vi "OSCILO.vi"(4 "Trigger Edge":u32, 5 "FIFO_SIZE":u32, 6 "SET":bool, 7 "TRIGGER_LEVEL":u32, 8 "error in (no error)":errorcluster, 9 "TRIG_DELAY":u32, 11 "TCP Network Connection in":refnum<k5>) -> (0 "error out":errorcluster, 2 "Oscilloscope":u32[](array[numeric]), 3 "TCP Network Connection out":refnum<k5>)   [LabVIEW 2019]
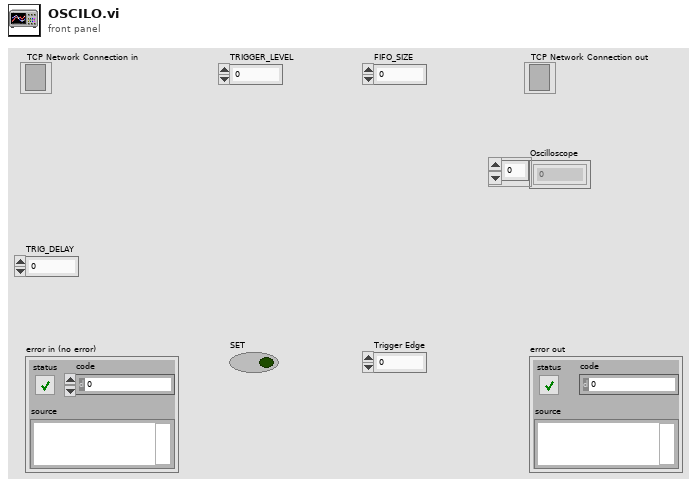
[diagram p1: front panel]
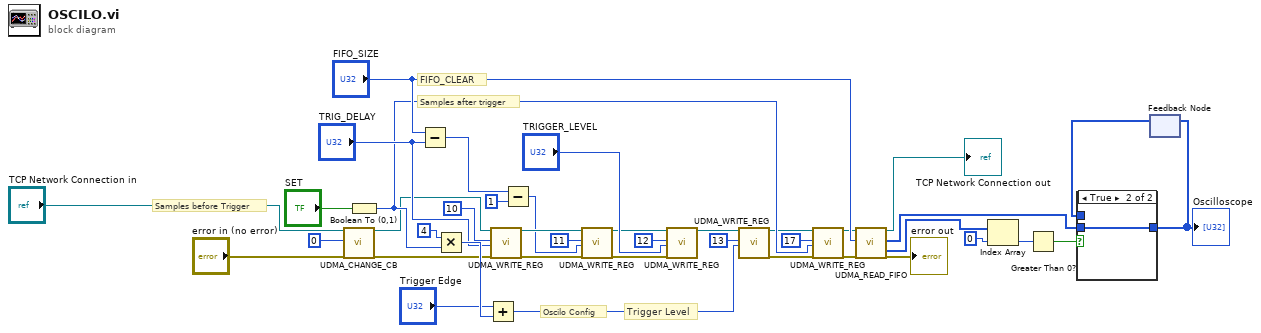
[diagram p0: block diagram]
diagram:
  # "FIFO_CLEAR"
  # "Oscilo Config"
  # "Trigger Level"
  # "Samples after trigger"
  # "Samples before Trigger"
  n1 = call "UDMA_CHANGE_CB.vi"("TCP Network Connection in"="TCP Network Connection in", "CB_ID"=u32 0, "error in (no error)"="error in (no error)") -> ("TCP Network Connection out"=w2:refnum<k5>, "error out"=w1:errorcluster)  [unwired: 14 in, 1 out]
  n2 = Boolean To (0,1)(Boolean="SET") -> (0, 1=w17:i16)
  n3 = Subtract(x="FIFO_SIZE", y="TRIG_DELAY") -> (x-y=w29:u32)
  n4 = Multiply(x=i16 4, y=w17) -> (x*y=w33:i16)
  n5 = Add(x="Trigger Edge", y=w33) -> (x+y=w26:u32)
  n6 = call "UDMA_WRITE_REG.vi"("TCP Network Connection in"=w2, "REG"=u32 10, "DATA"="TRIG_DELAY", "error in (no error)"=w1) -> ("TCP Network Connection out"=w32:refnum<k5>, "error out"=w31:errorcluster)  [unwired: 13 in, 1 out]
  n7 = Subtract(x=w29, y=u32 1) -> (x-y=w28:u32)
  n8 = call "UDMA_WRITE_REG.vi"("TCP Network Connection in"=w32, "REG"=u32 11, "DATA"=w28, "error in (no error)"=w31) -> ("TCP Network Connection out"=w23:refnum<k5>, "error out"=w22:errorcluster)  [unwired: 13 in, 1 out]
  n9 = call "UDMA_WRITE_REG.vi"("TCP Network Connection in"=w23, "REG"=u32 12, "DATA"="TRIGGER_LEVEL", "error in (no error)"=w22) -> ("TCP Network Connection out"=w24:refnum<k5>)  [unwired: 13 in, 2 out]
  n10 = call "UDMA_WRITE_REG.vi"("TCP Network Connection in"=w24, "REG"=u32 13, "DATA"=w26) -> ("TCP Network Connection out"=w15:refnum<k5>, "error out"=w16:errorcluster)  [unwired: 14 in, 1 out]
  n11 = call "UDMA_WRITE_REG.vi"("TCP Network Connection in"=w15, "REG"=u32 17, "DATA"=w17, "error in (no error)"=w16) -> ("TCP Network Connection out"=w14:refnum<k5>, "error out"=w13:errorcluster)  [unwired: 13 in, 1 out]
  n12 = call "UDMA_READ_FIFO.vi"("TCP Network Connection in"=w14, "N"="FIFO_SIZE", "error in (no error)"=w13) -> ("TCP Network Connection out"=→"TCP Network Connection out":refnum<k5>, "Oscilloscope"=w10:u32[], "Status"=w12:u8[], "error out"=→"error out":errorcluster)  [unwired: 13 in]
  n13 = Index Array(array=w12, index=0) -> (element=w6:u8)
  n14 = Greater Than 0?(x=w6) -> (x > 0?=w7:bool)
  n15 = feedback #1() -> (w9:u32[])  [unwired: 1 in]
  n16 = case shown="True" w7 {
    tunnel: [w41 w42] -> w8
    tunnel: w10 -> [_ w42]
    tunnel: w9 -> [w41 _]
    frame False {
    }
    frame True {
    }
  }
  "Oscilloscope" <- w8
  n17 = feedback-in #1(w8) -> ()
